vi "Autonomous A2 left-deliverswitch-move out of way.vi"   [LabVIEW 2017]
uses:
  Framework/Robot Global Data.vi
types:
  T1 = typedef "Command Status Info.ctl" = cluster{"Name":string, "Status":T2, "notifier out":T3}
  T2 = typedef "Completion Status.ctl" = enum16{"Successful", "Aborted", "Incomplete"}
  T3 = typedef "Completion Notifier.ctl" = refnum<notifier>
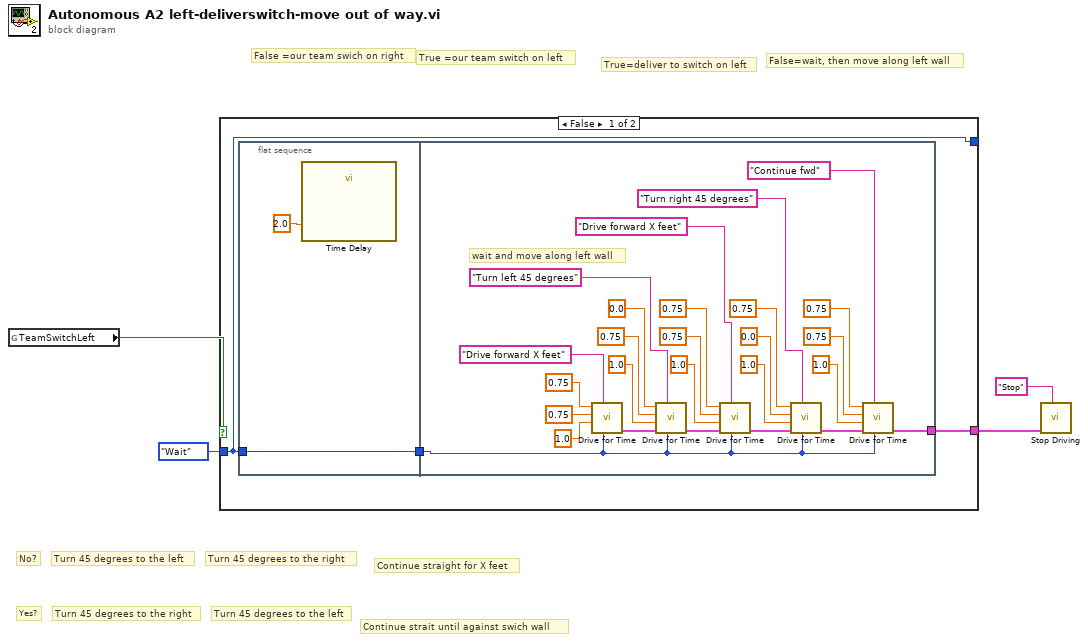
[diagram p0: block diagram]
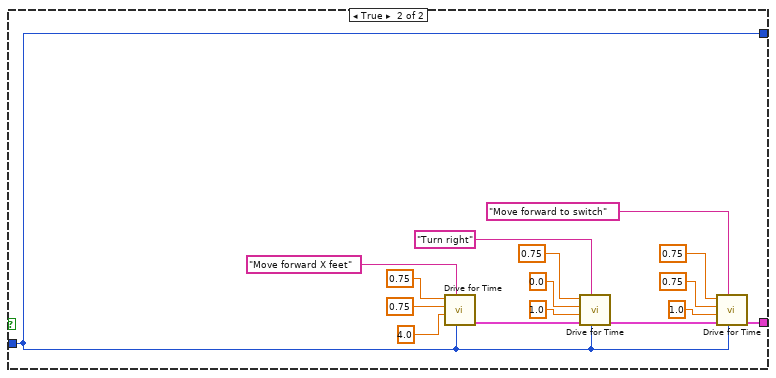
[diagram p2: hidden frame]
diagram:
  # "False=wait, then move along left wall"
  # "True=deliver to switch on left"
  # "False =our team swich on right"
  # "True =our team switch on left"
  # "Continue strait until against swich wall"
  # "Continue straight for X feet"
  # "Turn 45 degrees to the left"
  # "Turn 45 degrees to the right"
  # "Turn 45 degrees to the left"
  # "Turn 45 degrees to the right"
  # "No?"
  # "Yes?"
  n1 = global read "Robot Global Data.vi" "TeamSwitchLeft"() -> (w1:bool)
  n2 = case shown="False" w1 {
    tunnel: enum16{"Start", "Wait"}."Wait" ("Synchronication") -> [w6 w39]
    tunnel: [w7 w43] -> w2
    tunnel: [w6 w39] -> _
    frame False {
      n3 = flat-sequence {
        tunnel: w6 -> [w9]
        tunnel: [w9] -> w5
        tunnel: [w12] -> w7
        tunnel: w5 -> [w10]
        frame #0 {
          n4 = call "Time Delay"("Delay Time (s)"=2.0) -> ()  [unwired: 10 in, 1 out]
        }
        frame #1 {
          # "wait and move along left wall"
          n5 = call "Drive for Time.vi"("Synchronization"=w10, "Description"="Drive forward X feet", "Seconds"=1.0, "Right Speed"=0.75, "Left Speed"=0.75 ("Right Speed")) -> ("Command Info Out"=w28:T1)  [unwired: 5 in, 1 out]
          n6 = call "Drive for Time.vi"("Synchronization"=w10, "Description"="Turn left 45 degrees", "Command Info In"=w28, "Seconds"=1.0, "Right Speed"=0.75, "Left Speed"=0.0) -> ("Command Info Out"=w26:T1)  [unwired: 4 in, 1 out]
          n7 = call "Drive for Time.vi"("Synchronization"=w10, "Description"="Drive forward X feet", "Command Info In"=w26, "Seconds"=1.0, "Right Speed"=0.75, "Left Speed"=0.75 ("Right Speed")) -> ("Command Info Out"=w25:T1)  [unwired: 4 in, 1 out]
          n8 = call "Drive for Time.vi"("Synchronization"=w10, "Description"="Turn right 45 degrees", "Command Info In"=w25, "Seconds"=1.0, "Right Speed"=0.0, "Left Speed"=0.75) -> ("Command Info Out"=w13:T1)  [unwired: 4 in, 1 out]
          n9 = call "Drive for Time.vi"("Synchronization"=w10, "Description"="Continue fwd", "Command Info In"=w13, "Seconds"=1.0, "Right Speed"=0.75, "Left Speed"=0.75) -> ("Command Info Out"=w12:T1)  [unwired: 4 in, 1 out]
        }
      }
    }
    frame True {
      n10 = call "Drive for Time.vi"("Synchronization"=w39, "Description"="Move forward X feet", "Seconds"=4.0, "Right Speed"=0.75, "Left Speed"=0.75) -> ("Command Info Out"=w42:T1)  [unwired: 5 in, 1 out]
      n11 = call "Drive for Time.vi"("Synchronization"=w39, "Description"="Turn right", "Command Info In"=w42, "Seconds"=1.0, "Right Speed"=0.0, "Left Speed"=0.75) -> ("Command Info Out"=w41:T1)  [unwired: 4 in, 1 out]
      n12 = call "Drive for Time.vi"("Synchronization"=w39, "Description"="Move forward to switch", "Command Info In"=w41, "Seconds"=1.0, "Right Speed"=0.75, "Left Speed"=0.75) -> ("Command Info Out"=w43:T1)  [unwired: 4 in, 1 out]
    }
  }
  n13 = call "Stop Driving.vi"("Description"="Stop", "Command Info In"=w2) -> ()  [unwired: 9 in, 1 out]
